vi "Close project.vi"() -> ()   [LabVIEW 2026]
uses:
  <vilib>/Utility/error.llb/DialogType.ctl
panel:
  in  "Path":path
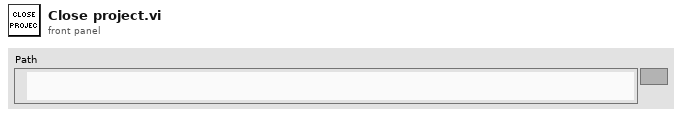
[diagram p1: front panel]
types:
  T1 = typedef "DialogType.ctl" = u16
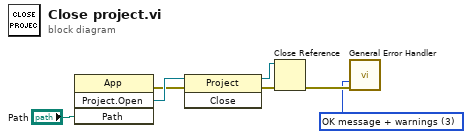
[diagram p0: block diagram]
diagram:
  w1 = T1 3 items=["no dialog", "OK message", "continue or stop message", "OK message + warnings", "continue/stop + warnings"] ("type of dialog (OK msg:1)")
  n1 = invoke class="App" method="Project.Open"("Path"="Path") -> (error out=w3:errorcluster, "Project:Open"=w4:refnum<vi>)  [unwired: 3 in, 2 out]
  n2 = invoke class="Project" method="Close"(reference=w4, error in=w3) -> (reference out=w5:refnum<vi>, error out=w6:errorcluster)  [unwired: 1 in, 1 out]
  n3 = Close Reference(reference=w5, error in (no error)=w6) -> (error out=w2:errorcluster)
  n4 = call <vilib>:"General Error Handler.vi"("type of dialog (OK msg:1)"=w1, "error in (no error)"=w2) -> ()  [unwired: 9 in, 5 out]
